vi "HeaderTPos.vi"(11 "Trap Path":path) -> (3 "TPos File":refnum<file>)   [LabVIEW 2013]
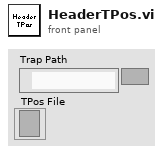
[diagram p1: front panel]
types:
  T1 = enum16{"big-endian, network order", "native, host order", "little-endian"}
  T2 = enum16{"open", "replace", "create", "open or create", "replace or create", "replace or create with confirmation"}
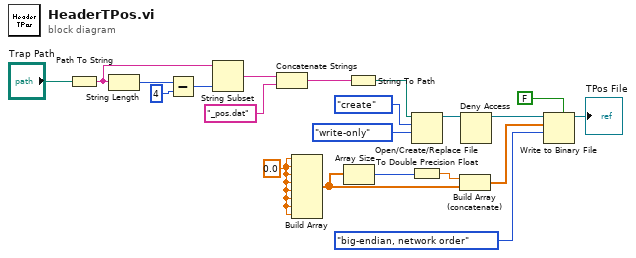
[diagram p0: block diagram]
diagram:
  w20 = 0.0 ("element")
  n1 = Path To String(path="Trap Path") -> (string=w2:string)
  n2 = String Length(string=w2) -> (length=w3:i32)
  n3 = Subtract(x=w3, y=4) -> (x-y=w5:i32)
  n4 = String Subset(string=w2, length (rest)=w5) -> (substring=w6:string)  [unwired: 1 out]
  n5 = Concatenate Strings(w6, "_pos.dat" ("string")) -> (w8:string)
  n6 = Build Array(w20, w20, w20, w20, w20, w20, w20, w20) -> (w19:dbl[])
  n7 = Array Size(array=w19) -> (size(s)=w17:i32)
  n8 = String To Path(string=w8) -> (path=w12:path)
  n9 = Open/Create/Replace File(file path (use dialog)=w12, operation (0:open)=T2."create", access (0:read/write)=enum16{"read/write", "read-only", "write-only"}."write-only") -> (refnum out=w11:refnum<file>)  [unwired: 1 in, 4 out]
  n10 = To Double Precision Float(number=w17) -> (double precision float=w18:dbl)
  n11 = Build Array (concatenate)(w18, w19) -> (w21:dbl[])
  n12 = Deny Access(7:w11) -> (3:w15:refnum<file>)  [unwired: 1 in, 2 out]
  n13 = Write to Binary File(file (use dialog)=w15, data=w21, 5:FALSE ("prepend array or string size? (T)"), 9:T1."big-endian, network order" ("byte order (0:big-endian, network order)")) -> (refnum out=→"TPos File":refnum<file>)  [unwired: 1 in, 3 out]
